vi "Check.vi"(8 "error in (no error)":errorcluster, 11 "FTPProtocol in":refnum<class "FTPProtocol.lvclass">) -> (0 "error out":errorcluster, 2 "Still alive?":bool, 3 "FTPProtocol out":refnum<class "FTPProtocol.lvclass">)   [LabVIEW 2020, in "FileSync -- FTP.lvlib" / "FTPProtocol.lvclass"]
uses:
  FTPProtocol.lvclass
  FTPProtocol.lvclass/FTPProtocol.ctl
  _support/FTP Toolkit/FTP Class/FTP.lvclass
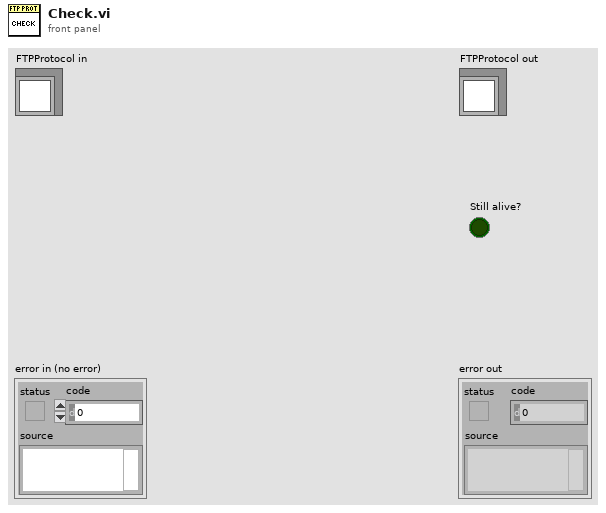
[diagram p1: front panel]
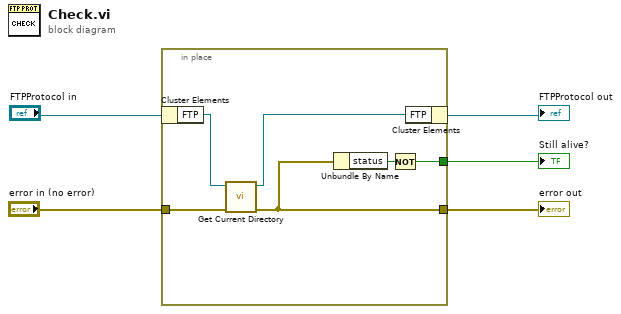
[diagram p0: block diagram]
diagram:
  n1 = in-place {
    in-place-border: "error in (no error)" -> [w11]
    in-place-border: [w8] -> w4
    in-place-border: [w6] -> w1
    n2 = in-place-cluster #1("FTPProtocol in") -> ("FTP"=w10:refnum<class "FTP.lvclass">)
    n3 = call "Get Current Directory.vi"("error in (no error)"=w11, "FTP in"=w10) -> ("error out"=w8:errorcluster, "FTP out"=w9:refnum<class "FTP.lvclass">)  [unwired: 7 in, 1 out]
    n4 = Unbundle By Name(w8) -> ("status"=w7:bool)
    n5 = Not(x=w7) -> (.not. x?=w6:bool)
    n6 = in-place-cluster #1("FTP"=w9) -> (→"FTPProtocol out":refnum<class "FTPProtocol.lvclass">)
  }
  "error out" <- w4
  "Still alive?" <- w1
